vi "ManualPanel_FISH02.vi"() -> ()   [LabVIEW 2019]
uses:
  device/device_global.vi
  device/ST_RMDS.llb/RMDS.lvclass
  device/TETECH_TC720.llb/TC720.lvclass
panel:
  in  "2":bool caption="1"
  in  "x":dbl
  in  "1":bool
  in  "SP_PUSH":bool
  in  "Vol(uL) 2":dbl
  in  "Speed(uL/s) 2":dbl
  in  "Execute":bool
  in  "SCAN Command":string
  in  "0":bool caption="1"
  in  "VICI Valve 2":i32(knob)=1 min=1 max=10 step=1 scale=1.0..10.0
  in  "VICI Valve":i32(knob)=1 min=1 max=10 step=1 scale=1.0..10.0
  in  "PP_STOP":bool
  in  "PP_WC":bool
  in  "SP_WC 2":bool
  out "I":bool
  in  "SP_IN":bool
  out "O":bool
  in  "SP_O":bool
  in  "SP_STOP":bool
  in  "SP_WC":bool
  in  "SP_PULL":bool
  in  "Vol(uL)":dbl
  in  "Speed(uL/s)":dbl
  in  "SP_RESET":bool
  in  "HOME Y":bool
  out "information":string
  in  "HOME X":bool
  in  "SUO":bool
  out "Execution Return":errorcluster
  out "Command Error":errorcluster
  out "Current Command Return":string
  in  "AUTOFOCUS":bool
  out "Current Command":string
  in  "PP_Out":bool
  in  "PP_In":bool
  in  "TC_OUTPUT":bool
  out "TC_GET":dbl=22.8
  in  "TC_SET":dbl=20.0
  out "Waveform Chart":dynamicdata(graph)=[{"t0"=timestamp(3646258585.695117 s since 1904-01-01), "dt"=1.0, "Y"=[23.03]}, {"t0"=timestamp(3646258585.664063 s since 1904-01-01), "dt"=1.0, "Y"=[22.8]}, {"t0"=timestamp(3646258585.664063 s since 1904-01-01), "dt"=1.0, "Y"=[10.0]}]
  # "waste"
  # "To waste"
  # "From Chip"
  # "Bypass"
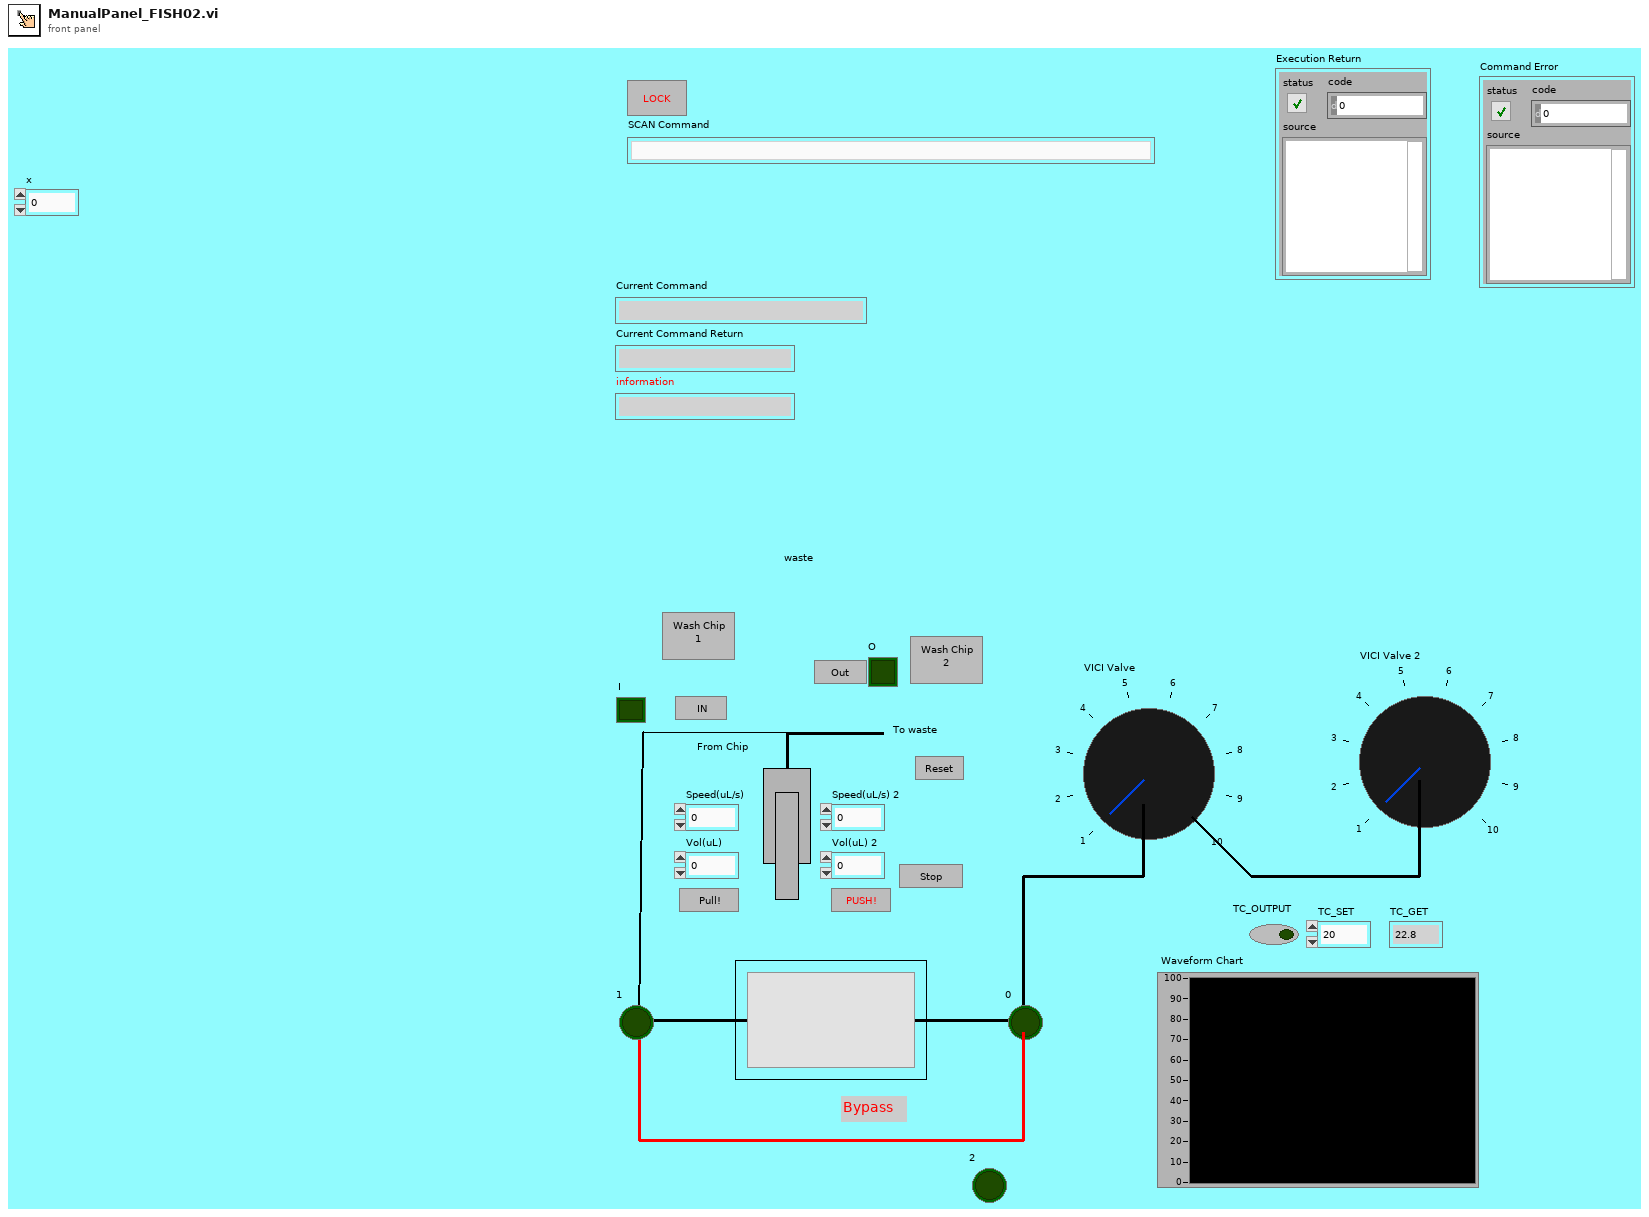
[diagram p1: front panel]
types:
  T1 = enum16{"open", "replace", "create", "open or create", "replace or create", "replace or create with confirmation"}
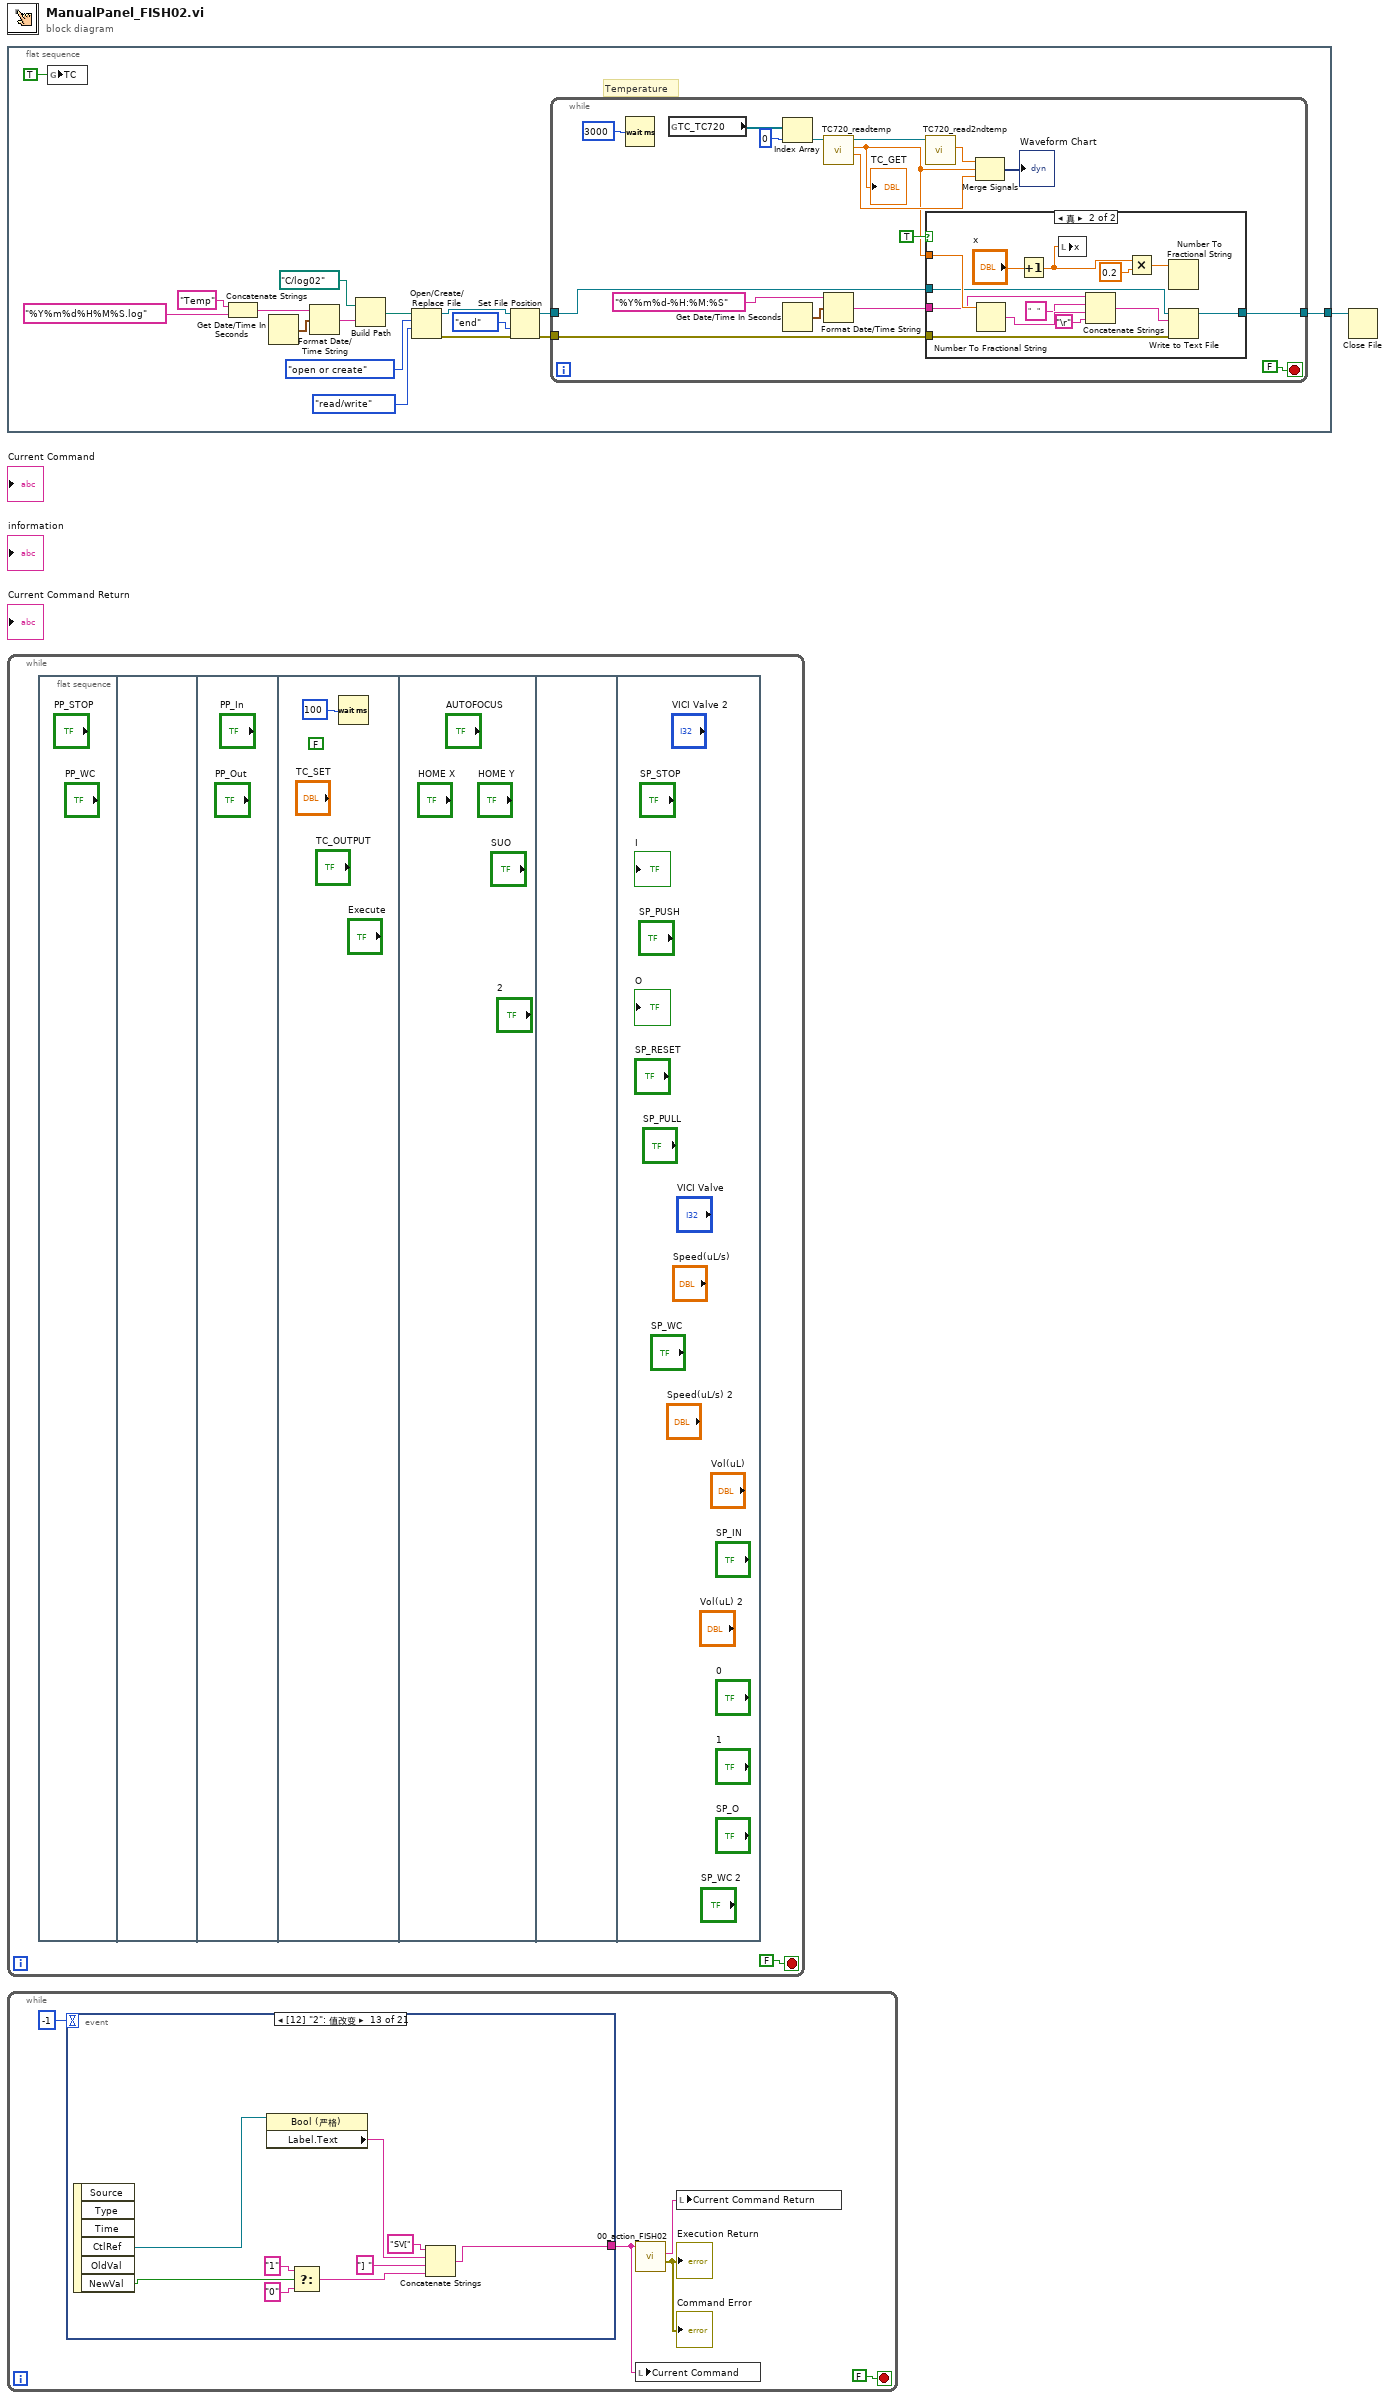
[diagram p0: block diagram]
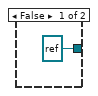
[diagram p2: hidden frame]
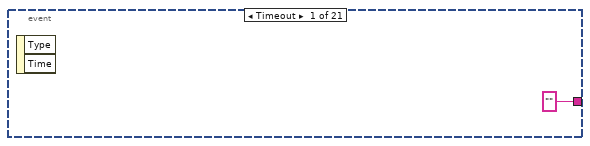
[diagram p3: hidden frame]
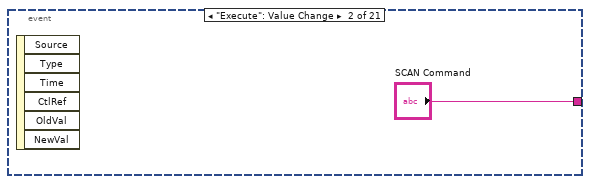
[diagram p4: hidden frame]
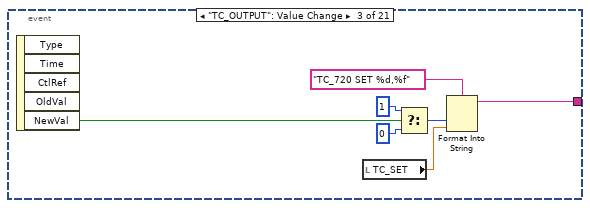
[diagram p5: hidden frame]
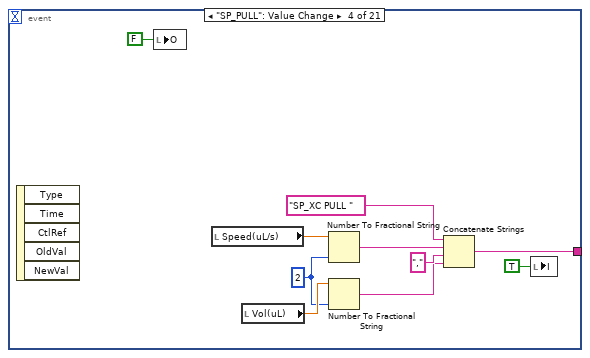
[diagram p6: hidden frame]
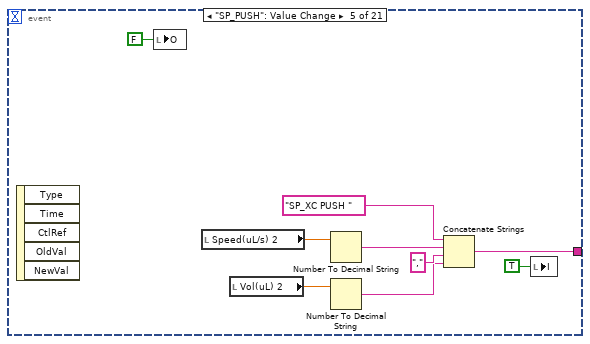
[diagram p7: hidden frame]
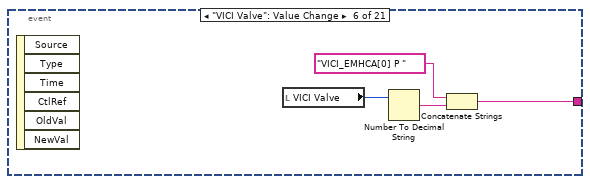
[diagram p8: hidden frame]
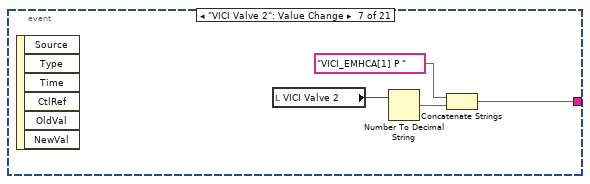
[diagram p9: hidden frame]
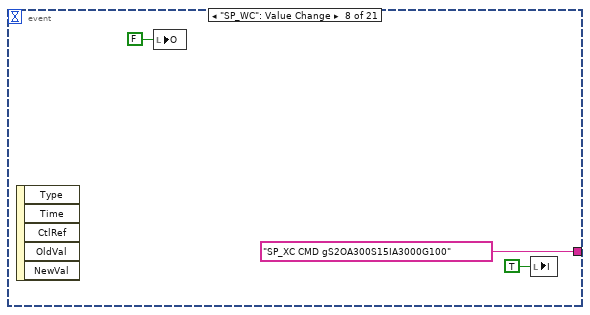
[diagram p10: hidden frame]
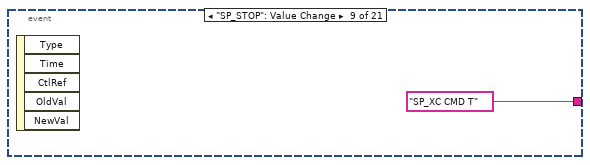
[diagram p11: hidden frame]
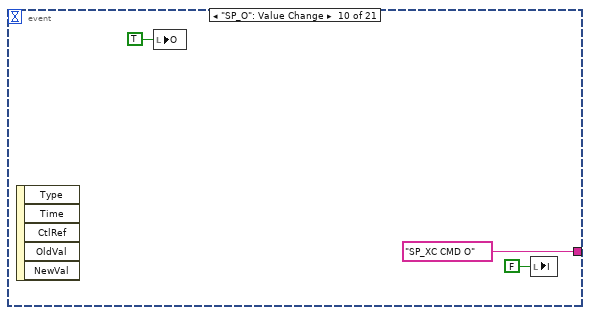
[diagram p12: hidden frame]
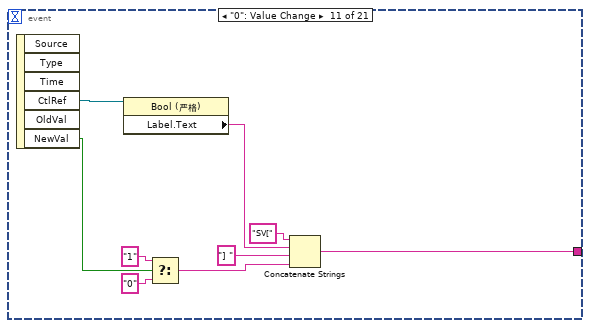
[diagram p13: hidden frame]
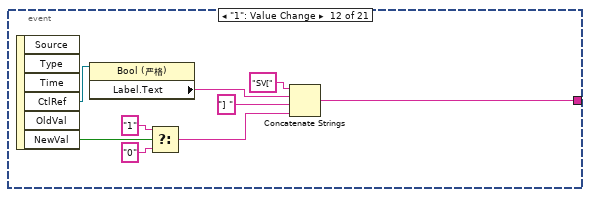
[diagram p14: hidden frame]
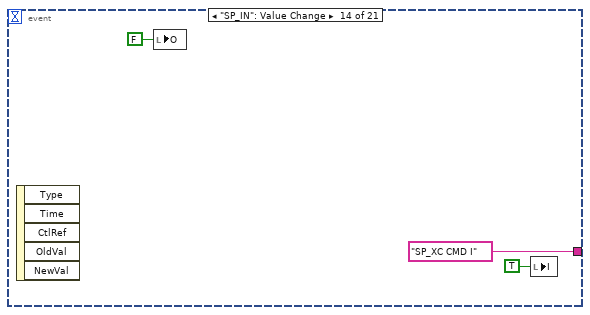
[diagram p15: hidden frame]
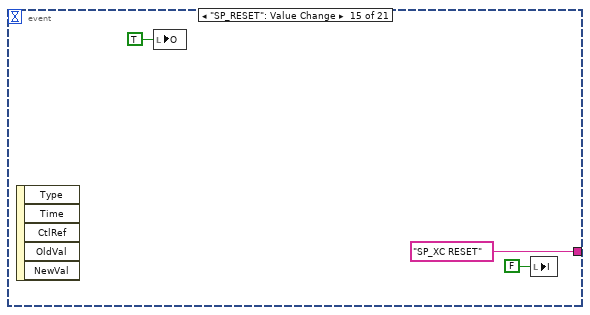
[diagram p16: hidden frame]
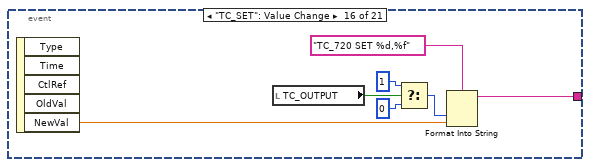
[diagram p17: hidden frame]
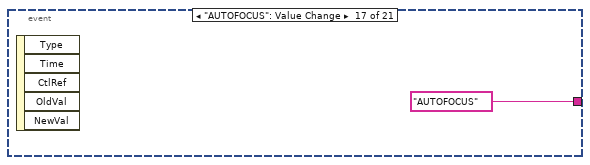
[diagram p18: hidden frame]
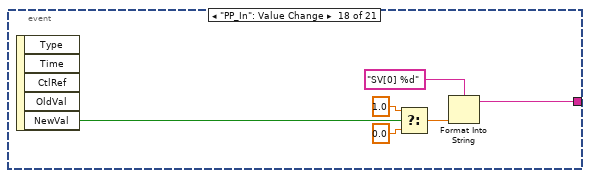
[diagram p19: hidden frame]
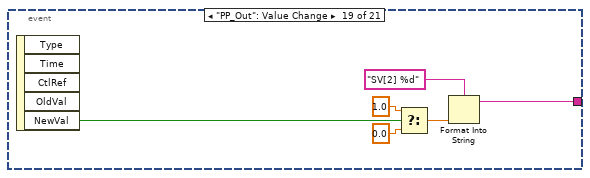
[diagram p20: hidden frame]
diagram:
  n1 = flat-sequence {
    tunnel: [w2] -> w1
    frame #0 {
      # "Temperature"
      n2 = global write "device_global.vi" "TC"(TRUE ("TC")) -> ()
      n3 = Concatenate Strings("Temp" ("string"), "%Y%m%d%H%M%S.log" ("time format string (%c)")) -> (w15:string)
      n4 = Get Date/Time In Seconds() -> (seconds since 1Jan1904=w14:timestamp)
      n5 = Format Date/Time String(time format string (%c)=w15, seconds (now)=w14) -> (date/time string=w5:string)  [unwired: 1 in]
      n6 = Build Path(base path=path "C:/log02" ("file path (use dialog)"), name or relative path=w5) -> (appended path=w7:path)
      n7 = Open/Create/Replace File(file path (use dialog)=w7, operation (0:open)=T1."open or create", access (0:read/write)=enum16{"read/write", "read-only", "write-only"}."read/write") -> (refnum out=w9:refnum<file>, error out=w8:errorcluster)  [unwired: 3 in, 1 out]
      n8 = Set File Position(refnum=w9, from (0:start)=enum16{"start", "end", "current"}."end", error in=w8) -> (refnum out=w4:refnum<file>, error out=w3:errorcluster)  [unwired: 1 in]
      n9 = while {
        tunnel: w4 -> [w21]
        tunnel: w3 -> [w20]
        tunnel: [w18] -> w2
        stop <- FALSE stop-if-true
        n10 = Wait (ms)(milliseconds to wait=i64 3000 ("Period")) -> ()  [unwired: 1 out]
        n11 = global read "device_global.vi" "TC_TC720"() -> (w34:refnum<class "TC720.lvclass">[])
        n12 = Index Array(array=w34, index=0) -> (element=w32:refnum<class "TC720.lvclass">)
        n13 = Get Date/Time In Seconds() -> (seconds since 1Jan1904=w23:timestamp)
        n14 = call-dynamic "TC720_readtemp.vi"("TC720 in"=w32) -> ("temp1set"=w30:dbl, "temp1get"=w19:dbl, "TC720 out"=w28:refnum<class "TC720.lvclass">)  [unwired: 6 in, 2 out]
        "TC_GET" <- w19
        n15 = Format Date/Time String(time format string (%c)="%Y%m%d-%H:%M:%S", seconds (now)=w23) -> (date/time string=w24:string)  [unwired: 1 in]
        n16 = call-dynamic "TC720_read2ndtemp.vi"("TC720 in"=w28) -> ("temp2get"=w29:dbl)  [unwired: 6 in, 4 out]
        n17 = case shown="真" TRUE {
          tunnel: [refnum<file> refnum ("refnum out") w46] -> w18
          tunnel: w19 -> [_ w45]
          tunnel: w24 -> [_ w38]
          tunnel: w21 -> [_ w37]
          tunnel: w20 -> [_ w36]
          frame False {
          }
          frame True {
            n18 = Number To Fractional String(number=w45) -> (F-format string=w48:string)  [unwired: 3 in]
            n19 = Increment(x="x") -> (x+1=w42:dbl)
            n20 = local write "x"(w42) -> ()
            n21 = Concatenate Strings(w38, "   " ("string"), w48, "\r") -> (w44:string)
            n22 = Multiply(x=w42, y=0.2) -> (x*y=w40:dbl)
            n23 = Number To Fractional String(number=w40) -> ()  [unwired: 3 in, 1 out]
            n24 = Write to Text File(file (use dialog)=w37, text=w44, error in=w36) -> (refnum out=w46:refnum<file>)  [unwired: 1 in, 2 out]
          }
        }
        n25 = Merge Signals(w29, w19, w30) -> (→"Waveform Chart":dynamicdata)
      }
    }
  }
  n26 = while {
    stop <- FALSE stop-if-true
    n27 = flat-sequence {
      frame #0 {
      }
      frame #1 {
      }
      frame #2 {
      }
      frame #3 {
        (unwired) FALSE
        n28 = Wait (ms)(milliseconds to wait=u32 100) -> ()  [unwired: 1 out]
      }
      frame #4 {
      }
      frame #5 {
      }
      frame #6 {
      }
    }
  }
  n29 = while {
    stop <- FALSE stop-if-true
    n30 = event shown="[12] \"2\": 值改变" {
      selector: _ -> [_ _ _ _ _ _ _ _ _ _ _ _ _ _ _ _ _ _ _ _ _]
      dyn-events: _ -> [_ _ _ _ _ _ _ _ _ _ _ _ _ _ _ _ _ _ _ _ _]
      timeout: -1 -> [_ _ _ _ _ _ _ _ _ _ _ _ _ _ _ _ _ _ _ _ _]
      tunnel: ["" ("Line") "SCAN Command" w58 w70 w75 w86 w88 "SP_XC CMD gS2OA300S15IA3000G100" ("format string") "SP_XC CMD T" ("format string") "SP_XC CMD O" ("format string") w99 w108 w119 "SP_XC CMD I" ("format string") "SP_XC RESET" ("format string") w132 "AUTOFOCUS" ("Line") w140 w146 _ w161] -> w53
      event Timeout {
        n31 = event-data() -> ()  [unwired: 1 in, 2 out]
      }
      event "Execute": Value Change {
        n32 = event-data() -> ()  [unwired: 1 in, 6 out]
      }
      event "TC_OUTPUT": Value Change {
        n33 = event-data() -> ("NewVal"=w59:bool)  [unwired: 1 in, 4 out]
        n34 = local read "TC_SET"() -> (w60:dbl)
        n35 = Select(t=1, s=w59, f=0) -> (s? t:f=w61:i32)
        n36 = Format Into String(format string="TC_720 SET %d,%f", w61, w60) -> (resulting string=w58:string)  [unwired: 2 in, 1 out]
      }
      event "SP_PULL": Value Change {
        w65 = i16 2 ("precision (6)")
        n37 = event-data() -> ()  [unwired: 1 in, 5 out]
        n38 = local write "O"(FALSE ("E")) -> ()
        n39 = local read "Speed(uL/s)"() -> (w68:dbl)
        n40 = local read "Vol(uL)"() -> (w69:dbl)
        n41 = Number To Fractional String(number=w68, precision (6)=w65) -> (F-format string=w67:string)  [unwired: 2 in]
        n42 = Number To Fractional String(number=w69, precision (6)=w65) -> (F-format string=w66:string)  [unwired: 2 in]
        n43 = Concatenate Strings("SP_XC PULL " ("string"), w67, "," ("string"), w66) -> (w70:string)
        n44 = local write "I"(TRUE ("I")) -> ()
      }
      event "SP_PUSH": Value Change {
        n45 = event-data() -> ()  [unwired: 1 in, 5 out]
        n46 = local write "O"(FALSE ("E")) -> ()
        n47 = local read "Speed(uL/s) 2"() -> (w80:dbl)
        n48 = local read "Vol(uL) 2"() -> (w81:dbl)
        n49 = Number To Decimal String(number=w80) -> (decimal integer string=w78:string)  [unwired: 1 in]
        n50 = Number To Decimal String(number=w81) -> (decimal integer string=w76:string)  [unwired: 1 in]
        n51 = Concatenate Strings("SP_XC PUSH " ("string"), w78, "," ("string"), w76) -> (w75:string)
        n52 = local write "I"(TRUE ("I")) -> ()
      }
      event "VICI Valve": Value Change {
        n53 = event-data() -> ()  [unwired: 1 in, 6 out]
        n54 = local read "VICI Valve"() -> (w85:i32)
        n55 = Number To Decimal String(number=w85) -> (decimal integer string=w84:string)  [unwired: 1 in]
        n56 = Concatenate Strings("VICI_EMHCA[0] P " ("Line"), w84) -> (w86:string)
      }
      event "VICI Valve 2": Value Change {
        n57 = event-data() -> ()  [unwired: 1 in, 6 out]
        n58 = local read "VICI Valve 2"() -> (w90:i32)
        n59 = Number To Decimal String(number=w90) -> (decimal integer string=w89:string)  [unwired: 1 in]
        n60 = Concatenate Strings("VICI_EMHCA[1] P " ("Line"), w89) -> (w88:string)
      }
      event "SP_WC": Value Change {
        n61 = event-data() -> ()  [unwired: 1 in, 5 out]
        n62 = local write "O"(FALSE ("E")) -> ()
        n63 = local write "I"(TRUE ("I")) -> ()
      }
      event "SP_STOP": Value Change {
        n64 = event-data() -> ()  [unwired: 1 in, 5 out]
      }
      event "SP_O": Value Change {
        n65 = event-data() -> ()  [unwired: 1 in, 5 out]
        n66 = local write "O"(TRUE ("E")) -> ()
        n67 = local write "I"(FALSE ("I")) -> ()
      }
      event "0": Value Change {
        n68 = event-data() -> ("CtlRef"=w101:refnum<vi>, "NewVal"=w100:bool)  [unwired: 1 in, 4 out]
        n69 = property class="Bool (严格)"(reference=w101) -> ("Label.Text"=w102:string)  [unwired: 1 in, 2 out]
        n70 = Select(t="1" ("format string"), s=w100, f="0" ("format string")) -> (s? t:f=w103:string)
        n71 = Concatenate Strings("SV[" ("format string"), w102, "] " ("string"), w103) -> (w99:string)
      }
      event "1": Value Change {
        n72 = event-data() -> ("CtlRef"=w109:refnum<vi>, "NewVal"=w110:bool)  [unwired: 1 in, 4 out]
        n73 = property class="Bool (严格)"(reference=w109) -> ("Label.Text"=w111:string)  [unwired: 1 in, 2 out]
        n74 = Select(t="1" ("format string"), s=w110, f="0" ("format string")) -> (s? t:f=w112:string)
        n75 = Concatenate Strings("SV[" ("format string"), w111, "] " ("string"), w112) -> (w108:string)
      }
      event "2": Value Change {
        n76 = event-data() -> ("CtlRef"=w117:refnum<vi>, "NewVal"=w118:bool)  [unwired: 1 in, 4 out]
        n77 = property class="Bool (严格)"(reference=w117) -> ("Label.Text"=w120:string)  [unwired: 1 in, 2 out]
        n78 = Select(t="1" ("format string"), s=w118, f="0" ("format string")) -> (s? t:f=w121:string)
        n79 = Concatenate Strings("SV[" ("format string"), w120, "] " ("string"), w121) -> (w119:string)
      }
      event "SP_IN": Value Change {
        n80 = event-data() -> ()  [unwired: 1 in, 5 out]
        n81 = local write "O"(FALSE ("E")) -> ()
        n82 = local write "I"(TRUE ("I")) -> ()
      }
      event "SP_RESET": Value Change {
        n83 = event-data() -> ()  [unwired: 1 in, 5 out]
        n84 = local write "O"(TRUE ("E")) -> ()
        n85 = local write "I"(FALSE ("I")) -> ()
      }
      event "TC_SET": Value Change {
        n86 = event-data() -> ("NewVal"=w133:dbl)  [unwired: 1 in, 4 out]
        n87 = local read "TC_OUTPUT"() -> (w137:bool)
        n88 = Select(t=1, s=w137, f=0) -> (s? t:f=w134:i32)
        n89 = Format Into String(format string="TC_720 SET %d,%f", w134, w133) -> (resulting string=w132:string)  [unwired: 2 in, 1 out]
      }
      event "AUTOFOCUS": Value Change {
        n90 = event-data() -> ()  [unwired: 1 in, 5 out]
      }
      event "PP_In": Value Change {
        n91 = event-data() -> ("NewVal"=w144:bool)  [unwired: 1 in, 4 out]
        n92 = Select(t=1.0, s=w144, f=0.0) -> (s? t:f=w143:dbl)
        n93 = Format Into String(format string="SV[0] %d" ("Line"), w143) -> (resulting string=w140:string)  [unwired: 2 in, 1 out]
      }
      event "PP_Out": Value Change {
        n94 = event-data() -> ("NewVal"=w150:bool)  [unwired: 1 in, 4 out]
        n95 = Select(t=1.0, s=w150, f=0.0) -> (s? t:f=w149:dbl)
        n96 = Format Into String(format string="SV[2] %d" ("Line"), w149) -> (resulting string=w146:string)  [unwired: 2 in, 1 out]
      }
      event "SUO": Value Change {
        n97 = event-data() -> ()  [unwired: 1 in, 5 out]
        n98 = global read "device_global.vi" "RMDS"() -> (w156:refnum<class "RMDS.lvclass">[])
        n99 = Index Array(array=w156, index=1) -> (element=w155:refnum<class "RMDS.lvclass">)
        n100 = Index Array(array=w156, index=0) -> (element=w152:refnum<class "RMDS.lvclass">)
        n101 = call-dynamic "RMDS_init.vi"("COM PORT"=refnum<visa-resource-name> "COM8", "RMDS in"=w155) -> ()  [unwired: 8 in, 2 out]
        n102 = call-dynamic "RMDS_init.vi"("COM PORT"=refnum<visa-resource-name> "COM7", "RMDS in"=w152) -> ()  [unwired: 8 in, 2 out]
      }
      event "HOME X": Value Change {
        n103 = event-data() -> ()  [unwired: 1 in, 5 out]
        n104 = Format Into String(initial string="ST_ADV MOVA " ("format string"), 0.0 ("input 1"), 0.0 ("input 2")) -> (resulting string=w161:string)  [unwired: 2 in, 1 out]
      }
    }
    n105 = call "00_action_FISH02.vi"("Line"=w53) -> ("Execution Return"=→"Command Error" →"Execution Return":errorcluster, "Return"=w52:string)  [unwired: 7 in, 2 out]
    n106 = local write "Current Command"(w53) -> ()
    n107 = local write "Current Command Return"(w52) -> ()
  }
  n108 = Close File(refnum=w1) -> ()  [unwired: 1 in, 2 out]
